vi "Send_Command_Ref.vi"(8 "error in":errorcluster, 10 "command":string="PING", 11 "refnum in":refnum<vi>) -> (0 "error out":errorcluster, 2 "Data":T1)   [LabVIEW 2020]
uses:
  SubVIs/Controls/redis-data.ctl
  SubVIs/Controls/redis-type.ctl
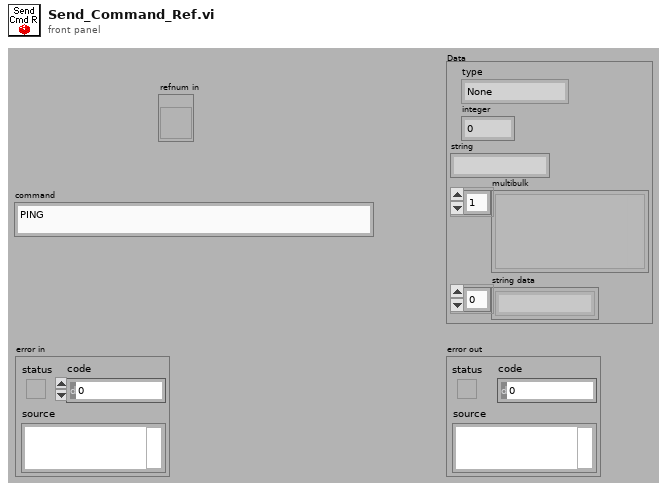
[diagram p1: front panel]
types:
  T1 = typedef "redis-data.ctl" = cluster{"type":enum16{"None", "Error", "Status", "Nil", "Integer", "String", "Multibulk"}, "integer":i64, "string":string, "multibulk":variant[], "string data":string[]}
  T2 = typedef "redis-type.ctl" = enum16{"None", "Error", "Status", "Nil", "Integer", "String", "Multibulk"}
  T3 = cluster{"integer":i64, "string":string, "multibulk":variant[]}
  T4 = typedef "redis-reply.ctl" = cluster{"integer":i64, "string":string, "multibulk":variant[]}
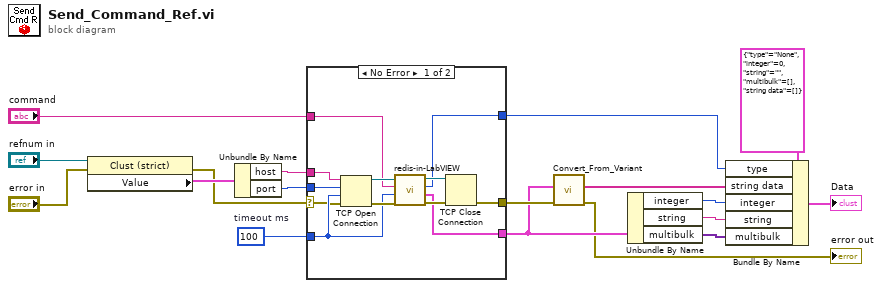
[diagram p0: block diagram]
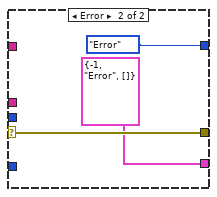
[diagram p2: hidden frame]
diagram:
  w18 = 100  # timeout ms
  n1 = property class="Clust (strict)"(reference="refnum in", error in="error in") -> (error out=w12:errorcluster, "Value"=w17:cluster{"host":string, "port":u16})  [unwired: 1 out]
  n2 = Unbundle By Name(w17) -> ("host"=w16:string, "port"=w15:u16)
  n3 = case shown="No Error" w12 {
    selector: w12 -> [w20 w33]
    tunnel: w15 -> [w30 _]
    tunnel: [w28 redis-type."Error" ("reply type")] -> w10
    tunnel: [w19 T3 {"integer"=-1, "string"="Error", "multibulk"=[]} ("reply")] -> w3
    tunnel: w16 -> [w27 _]
    tunnel: [w25 w33] -> w4
    tunnel: w18 -> [w22 _]
    tunnel: "command" -> [w21 _]
    frame No Error {
      n4 = TCP Open Connection(address=w27, remote port or service name=w30, timeout ms (60000)=w22, error in (no error)=w20) -> (connection ID=w24:refnum<k5>, error out=w23:errorcluster)  [unwired: 1 in]
      n5 = call "redis-in-LabVIEW.vi"("Error in"=w23, "Timeout ms"=w22, "Command"=w21, "TCP in"=w24) -> ("Error out"=w26:errorcluster, "redis reply"=w19:T4, "reply type"=w28:T2, "TCP out"=w29:refnum<k5>)
      n6 = TCP Close Connection(connection ID=w29, error in (no error)=w26) -> (error out=w25:errorcluster)  [unwired: 1 in, 1 out]
    }
    frame Error {
    }
  }
  n7 = call "Convert_From_Variant.vi"("error in"=w4, "Data in"=w3) -> ("error out"=→"error out":errorcluster, "String data out"=w1:string[])  [unwired: 8 in]
  n8 = Unbundle By Name(w3) -> ("integer"=w9:i64, "string"=w8:string, "multibulk"=w7:variant[])
  n9 = Bundle By Name(cluster=T1 {"type"=enum."None", "integer"=0, "string"="", "multibulk"=[], "string data"=[]} ("Data"), "type"=w10, "string data"=w1, "integer"=w9, "string"=w8, "multibulk"=w7) -> (→"Data":T1)
